vi "UT_006_LV to TMOL.vi"() -> ()   [LabVIEW 2017]
uses:
  4ff207aa-191a-44af-8f7a-4e6e6b751422.vi
  <vilib>/addons/_JKI Toolkits/Caraya/classes/Assert/Assert True.vi
  lib/TOML to LabVIEW.vi
  <vilib>/addons/_JKI Toolkits/Caraya/classes/Assert/Assert Almost Equal_Float.vi
  <vilib>/addons/_JKI Toolkits/Caraya/classes/Test/Test.lvclass
  lib/TOML.lvlib
  <vilib>/addons/_JKI Toolkits/Caraya/classes/Assert/Assert.lvclass
panel:
  out "Cluster 2":T1={"2d-array-string"=[["a", "b", "c"], ["d", "e", "f"], ["g", "h", "i"]], "1d-array-float"=[3.14, nan, 1.123], "sub-cluster"={"string"="hello world", "path"=path "C:/dev/GitHub/.gitignore"}, "timestamp"=timestamp(3701448577.464638 s since 1904-01-01), "1d-array-cluster"=[{"string"="one", "int"=1}, {"string"="five", "int"=5}]}
  out "error out 2":errorcluster
  out "String":string
  in  "Cluster":T1={"2d-array-string"=[["a", "b", "c"], ["d", "e", "f"], ["g", "h", "i"]], "1d-array-float"=[3.14, nan, 1.123], "sub-cluster"={"string"="hello world", "path"=path "C:/dev/GitHub/.gitignore"}, "timestamp"=timestamp(3701448577.47 s since 1904-01-01), "1d-array-cluster"=[{"string"="one", "int"=1}, {"string"="five", "int"=5}]}
  out "error out":errorcluster
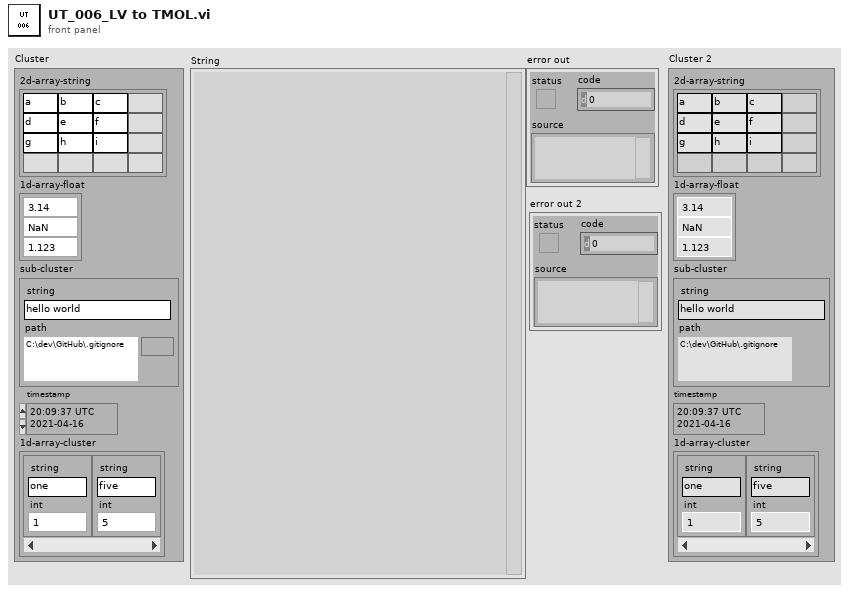
[diagram p1: front panel]
types:
  T1 = cluster{"2d-array-string":string[][], "1d-array-float":dbl[], "sub-cluster":cluster{"string":string, "path":path}, "timestamp":timestamp, "1d-array-cluster":cluster{"string":string, "int":i32}[]}
  T2 = typedef "TOML.lvlib/TOML Value.ctl" = cluster{"type":enum16{"Table", "Array", "String", "Integer", "Float", "Boolean", "Offset Date-Time", "Local Date-Time", "Local Date", "Local Time", "Path"}, "value":variant}
  T3 = cluster{"2d-array-string":bool[][], "1d-array-float":bool[], "sub-cluster":cluster{"string":bool, "path":bool}, "timestamp":bool, "1d-array-cluster":cluster{"string":bool, "int":bool}[]}
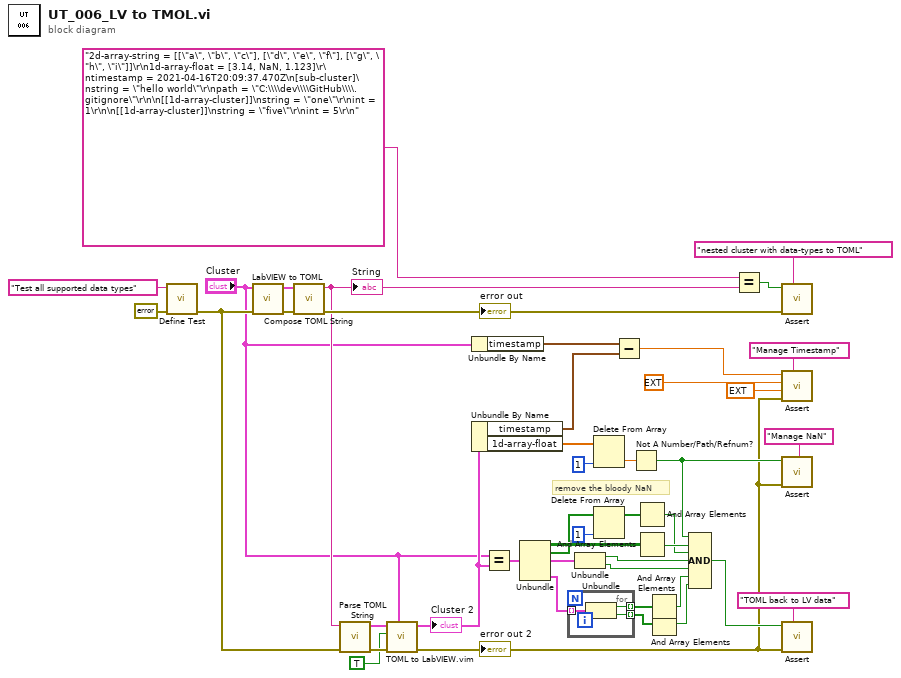
[diagram p0: block diagram]
diagram:
  # "remove the bloody NaN"
  n1 = call <vilib>:"Define Test.vi"("error in (no error)"=errorcluster {"status"=FALSE, "code"=0, "source"=""}, "Label (VI Title)"="Test all supported data types") -> ("error out"=w34:errorcluster)  [unwired: 9 in]
  n2 = call "LabVIEW to TOML.vi"("error in (no error)"=w34, "LV Value"="Cluster") -> ("error out"=w41:errorcluster, "TOML Value"=w33:T2)  [unwired: 8 in]
  n3 = call "Compose TOML String.vi"("error in (no error)"=w41, "Value"=w33) -> ("error out"=w40:errorcluster, "String"=w37:string)  [unwired: 8 in]
  "error out" <- w40
  "String" <- w37
  n4 = call "Parse TOML String.vi"("error in (no error)"=w34, "String"=w37) -> ("error out"=w38:errorcluster, "Value"=w32:T2)  [unwired: 8 in]
  n5 = call "TOML to LabVIEW.vim"("datatype"="Cluster", "error in (no error)"=w38, "Error if missing element"=TRUE, "Value"=w32) -> ("error out"=w5:errorcluster, "LV Data"=w15:T1)  [unwired: 5 in, 1 out]
  "error out 2" <- w5
  "Cluster 2" <- w15
  n6 = Unbundle By Name("Cluster") -> ("timestamp"=w9:timestamp)
  n7 = Unbundle By Name(w15) -> ("timestamp"=w3:timestamp, "1d-array-float"=w14:dbl[])
  n8 = Equal?(x="Cluster", y=w15) -> (x = y?=w30:T3)
  n9 = Unbundle(w30) -> ("2d-array-string"=w25:bool[][], "1d-array-float"=w19:bool[], "sub-cluster"=w29:cluster{"string":bool, "path":bool}, "1d-array-cluster"=w28:cluster{"string":bool, "int":bool}[])  [unwired: 1 out]
  n10 = for {
    tunnel: w28 -> [w47] mode=indexing
    tunnel: [w46] -> w23 mode=indexing
    tunnel: [w45] -> w22 mode=indexing
    n11 = Unbundle(w47) -> ("string"=w46:bool, "int"=w45:bool)
  }
  n12 = Unbundle(w29) -> ("string"=w27:bool, "path"=w26:bool)
  n13 = Delete From Array(array=w14, index=1) -> (deleted portion=w12:dbl)  [unwired: 1 in, 1 out]
  n14 = Delete From Array(array=w19, index=1) -> (array with subset deleted=w17:bool[])  [unwired: 1 in, 1 out]
  n15 = Subtract(x=w9, y=w3) -> (x-y=w4:dbl)
  n16 = Not A Number/Path/Refnum?(number/path/refnum=w12) -> (NaN/Path/Refnum?=w7:bool)
  n17 = And Array Elements(Boolean array=w17) -> (logical AND=w16:bool)
  n18 = And Array Elements(Boolean array=w25) -> (logical AND=w24:bool)
  n19 = And Array Elements(Boolean array=w23) -> (logical AND=w21:bool)
  n20 = And Array Elements(Boolean array=w22) -> (logical AND=w20:bool)
  n21 = Compound Arithmetic op=AND(w7, w24, w16, w27, w26, w21, w20) -> (w11:bool)
  n22 = Equal?(x="2d-array-string = [[\"a\", \"b\", \"c\"], [\"d\", \"e\", \"f\"], [\"g\", \"h\", \"i\"]]\r\n1d-array-float = [3.14, NaN, 1.123]\r\ntimestamp = 2021-04-16T20:09:37.470Z\n[sub-cluster]\nstring = \"hello world\"\r\npath = \"C:\\\\dev\\\\GitHub\\\\.gitignore\"\r\n\n[[1d-array-cluster]]\nstring = \"one\"\r\nint = 1\r\n\n[[1d-array-cluster]]\nstring = \"five\"\r\nint = 5\r\n", y=w37) -> (x = y?=w31:bool)
  n23 = call-poly <vilib>:"Assert.vi"("Label"="nested cluster with data-types to TOML" ("Label (VI Title)"), "error in (no error)"=w40, "True?"=w31) -> ()  [unwired: 8 in, 1 out]
  n24 = call-poly <vilib>:"Assert.vi"("Label"="Manage Timestamp" ("Label (VI Title)"), "error in (no error)"=w5, "Tolerance"=ext 0.00000100000000000000000004, "Y"=ext 0.0, "X"=w4) -> ()  [unwired: 6 in, 1 out]
  n25 = call-poly <vilib>:"Assert.vi"("Label"="Manage NaN" ("Label (VI Title)"), "error in (no error)"=w5, "True?"=w7) -> ()  [unwired: 8 in, 1 out]
  n26 = call-poly <vilib>:"Assert.vi"("Label"="TOML back to LV data" ("Label (VI Title)"), "error in (no error)"=w5, "True?"=w11) -> ()  [unwired: 8 in, 1 out]
